vi "loopStop.vi"(8 "error in (no error)":errorcluster, 11 "WinX32Camera in":refnum<class "WinX32Camera.lvclass">) -> (0 "error out":errorcluster, 3 "WinX32Camera out":refnum<class "WinX32Camera.lvclass">)   [LabVIEW 2011, in "WinX32Camera.lvclass"]
uses:
  WinX32Camera.lvclass
  WinX32Camera.lvclass/WinX32Camera.ctl
  PixelflySA/PixelflySA.lvclass
  Channels.lvlib
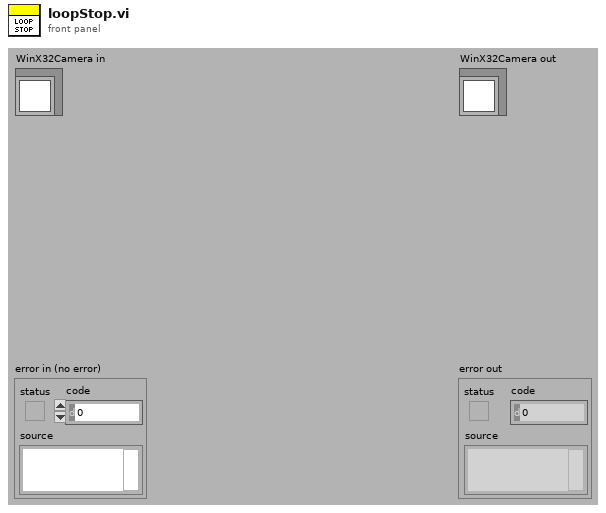
[diagram p1: front panel]
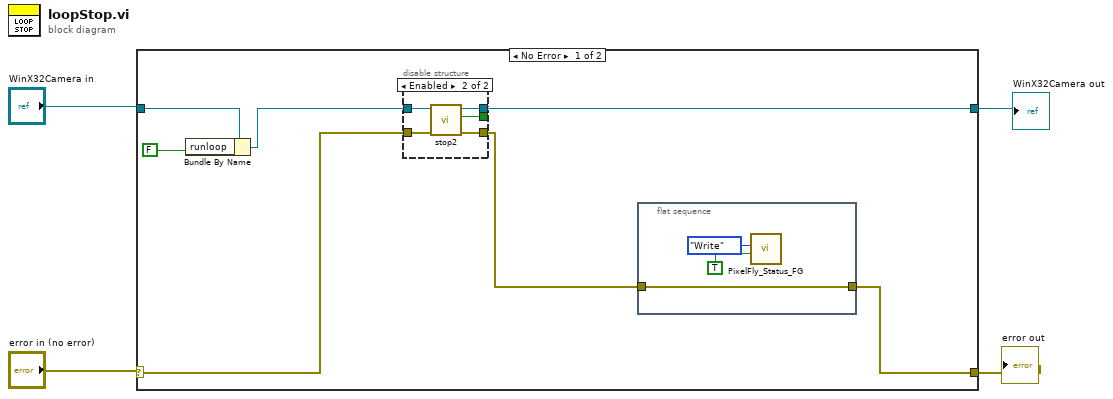
[diagram p0: block diagram]
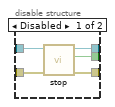
[diagram p2: hidden frame]
diagram:
  n1 = case shown="No Error" "error in (no error)" {
    selector: "error in (no error)" -> [w11 w26]
    tunnel: [w5 w26] -> w1
    tunnel: [w10 w25] -> w4
    tunnel: "WinX32Camera in" -> [w8 w25]
    frame No Error {
      n2 = Bundle By Name(cluster=w8, "runloop"=FALSE) -> (w7:refnum<class "WinX32Camera.lvclass">)
      n3 = disable-structure shown="Enabled" {
        disable-tunnel: w11 -> [w19 w21]
        disable-tunnel: [w18 w22] -> w6
        disable-tunnel: [w17 w20] -> _
        disable-tunnel: [w16 w23] -> w10
        disable-tunnel: w7 -> [w15 w24]
        frame Disabled {
          n4 = call-dynamic "stop.vi"("error in (no error)"=w19, "Pixelfly in"=w15) -> ("error out"=w18:errorcluster, "stopped?"=w17:bool, "Pixelfly out"=w16:refnum<class "PixelflySA.lvclass">)  [unwired: 6 in, 1 out]
        }
        frame Enabled {
          n5 = call "stop2.vi"("error in (no error)"=w21, "WinX32Camera in"=w24) -> ("error out"=w22:errorcluster, "stopped?"=w20:bool, "WinX32Camera out"=w23:refnum<class "WinX32Camera.lvclass">)  [unwired: 6 in, 1 out]
        }
      }
      n6 = flat-sequence {
        tunnel: w6 -> [w12]
        tunnel: [w12] -> w5
        frame #0 {
          n7 = call "PixelFly_Status_FG.vi"("stop"=TRUE, "Action"=enum16{"Write", "Read"}."Write") -> ()  [unwired: 9 in, 1 out]
        }
      }
    }
    frame Error {
    }
  }
  "error out" <- w1
  "WinX32Camera out" <- w4
